vi "Any to LabVIEW data.vi"(8 "error in":errorcluster, 10 "Data Order":T2(array[cluster]), 11 "Buffer":u8[](array[numeric])) -> (0 "error out":errorcluster, 2 "Output Data":T2(array[cluster]))   [LabVIEW 2020, in "Measurement Client Wrapper.lvclass"]
uses:
  Measurement Client Wrapper.lvclass
  <vilib>/TAF/LabVIEW Measurement Client/RPC Messages/ni_measurements_v1_Type.ctl
  <vilib>/gRPC/LabVIEW gRPC Library/Server API/typeDefs/Message Element Type.ctl
  ad0f9f6a-a690-4257-9139-53c7472e02e4.vi
  5e3468d2-7d53-449c-b4e1-cc5e8415f542.vi
  a6d26e38-1f9c-4531-8e6d-7eca794b9268.vi
  6111f2b2-3cd3-499d-ba70-c96985ac6ea8.vi
  21c55018-6bd1-46ad-94e2-895e688ed211.vi
  32480346-ebdd-43b9-a875-b6da9cef7217.vi
  4be456c1-ed59-4877-98ac-649a9044a973.vi
  e11fe247-09ff-4f5c-b897-2bd6ac17fb2f.vi
  e4b28d65-13ba-4e1e-8e9f-cbb4a39d886c.vi
  6b74e1a6-e30e-492b-a672-8f47ae6b4846.vi
  c7e14ed0-4c40-453e-98d2-21eea3b9c679.vi
  6e10cc60-964f-4e3c-a26b-7e2c601abf3f.vi
  4b20a9c0-4656-4d25-ac59-f75dc05d9fa7.vi
  999d58cf-c7d1-4a48-9a2f-662ae33a0057.vi
  b2ef58c8-55fb-46b3-8ffc-837df10363ae.vi
  811a2afd-07f9-4200-a7ec-155e2e775304.vi
  83b3a3de-e939-47b1-b683-bf64c49ab1e3.vi
  2e5f1bf6-8538-4323-9d72-f5ea1c9cc5e7.vi
  afd62ca2-246d-4ad4-bf5c-cd30e0a38d2e.vi
  b36e44fd-35bf-4184-b4fe-1327aa710fa9.vi
  613c056b-bfa0-4713-9fab-606e06d1fb15.vi
  d8424940-31d6-4816-8eab-b70d00974e91.vi
  0a60d30e-f22a-4deb-b9a9-4eb16321122e.vi
  430fb88b-afb0-4053-b427-f6628c3fec79.vi
  7ca7eab8-344c-48df-b026-809a17bb004d.vi
  89faac69-16e0-4e7e-99b5-b284c15014e6.vi
  e0a13140-8de5-47f3-97ec-5164ad61690d.vi
  32ddbda6-5255-4a5b-8b1b-da880a53ef98.vi
  20ed89fe-5e49-4e0f-9c89-ad84795baeb7.vi
  a81d3560-aafc-4ad9-a891-7c5845250d01.vi
  9ad9bf5a-c2fa-470e-917f-71ccee8fcf23.vi
  b78f8f4b-0643-45f3-92be-5419717043af.vi
  e0daed00-c2e0-4d52-9c25-0b8676dbe675.vi
  <vilib>/gRPC/LabVIEW gRPC Library/Server API/Server/Get Server DLL Path.vi
  <vilib>/gRPC/LabVIEW gRPC Library/gprc-lvsupport-release.lvlib
  <vilib>/TAF/LabVIEW Measurement Client/Measurement_client-release.lvlib
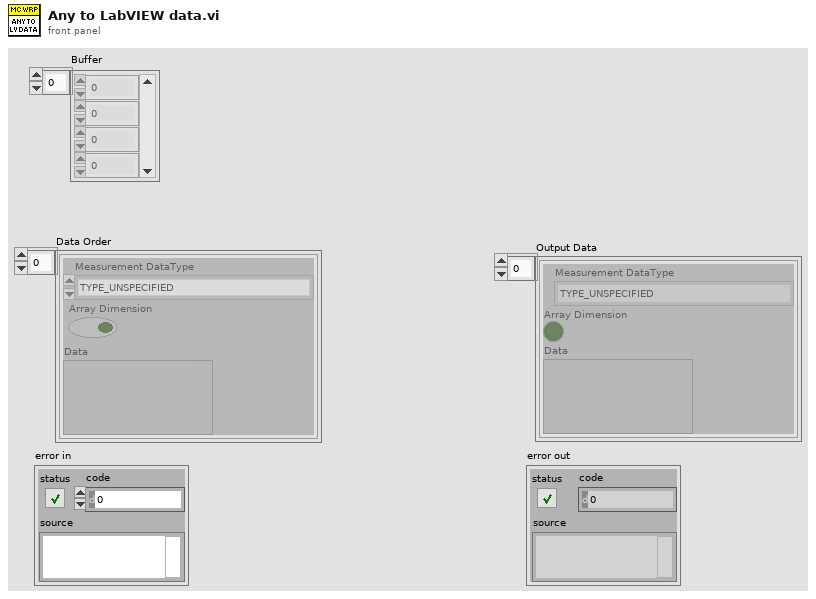
[diagram p1: front panel]
types:
  T1 = typedef "Measurement_client-release.lvlib/ni_measurements_v1_Type.ctl" = enum32{"TYPE_UNSPECIFIED", "TYPE_DOUBLE", "TYPE_FLOAT", "TYPE_INT64", "TYPE_UINT64", "TYPE_INT32", "TYPE_FIXED64", "TYPE_FIXED32", "TYPE_BOOL", "TYPE_STRING", "TYPE_GROUP", "TYPE_MESSAGE", "TYPE_BYTES", "TYPE_UINT32", "TYPE_ENUM", "TYPE_SFIXED32", "TYPE_SFIXED64", "TYPE_SINT32", "TYPE_SINT64"}
  T2 = cluster{"Measurement DataType":T1, "Array Dimension":bool, "Data":variant}[]
  T3 = typedef "gprc-lvsupport-release.lvlib/grpcId.ctl" = u64
  T4 = typedef "gprc-lvsupport-release.lvlib/Message Element Type.ctl" = enum32{"Int32Value", "FloatValue", "DoubleValue", "BoolValue", "StringValue", "MessageValue", "Int64Value", "UInt32Value", "UInt64Value", "EnumValue", "Bytes", "Fixed64", "Fixed32", "SFixed64", "SFixed32", "SInt64", "SInt32"}
  T5 = cluster{"Measurement DataType":T1, "Array Dimension":bool, "Data":variant}
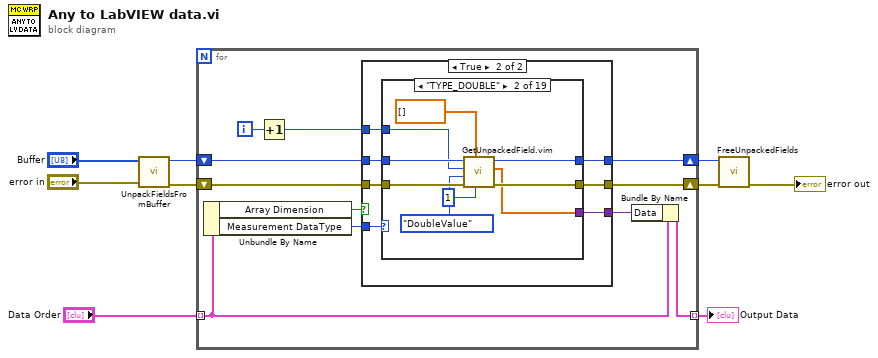
[diagram p0: block diagram]
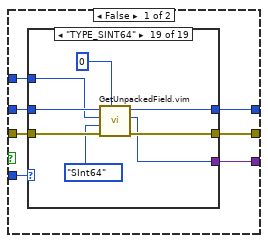
[diagram p2: hidden frame]
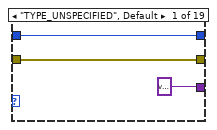
[diagram p3: hidden frame]
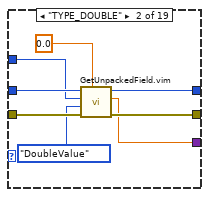
[diagram p4: hidden frame]
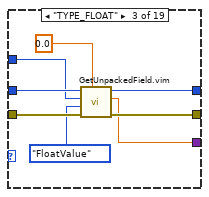
[diagram p5: hidden frame]
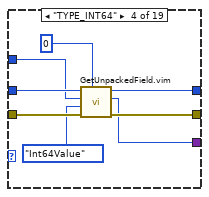
[diagram p6: hidden frame]
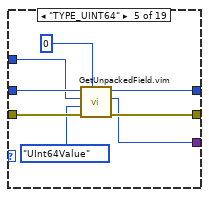
[diagram p7: hidden frame]
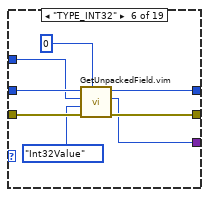
[diagram p8: hidden frame]
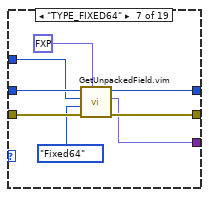
[diagram p9: hidden frame]
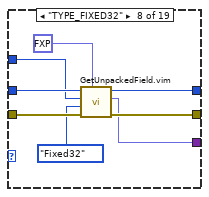
[diagram p10: hidden frame]
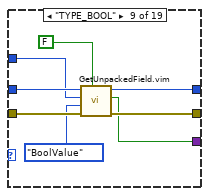
[diagram p11: hidden frame]
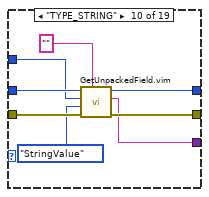
[diagram p12: hidden frame]
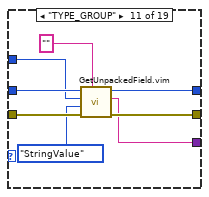
[diagram p13: hidden frame]
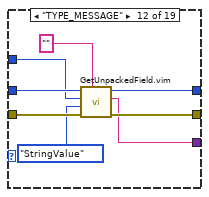
[diagram p14: hidden frame]
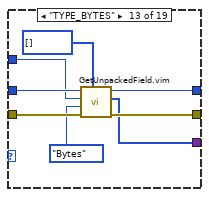
[diagram p15: hidden frame]
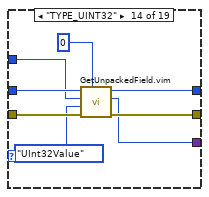
[diagram p16: hidden frame]
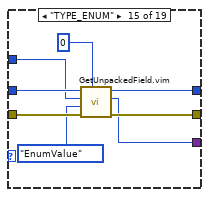
[diagram p17: hidden frame]
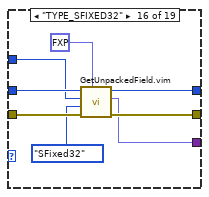
[diagram p18: hidden frame]
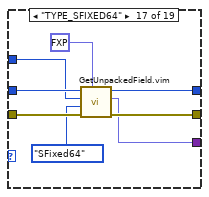
[diagram p19: hidden frame]
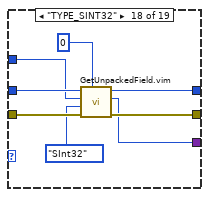
[diagram p20: hidden frame]
diagram:
  n1 = call <vilib>:"UnpackFieldsFromBuffer.vi"("error in (no error)"="error in", "Buffer"="Buffer") -> ("error out"=w8:errorcluster, "Fields Ref Out"=w9:T3)  [unwired: 8 in]
  n2 = for {
    tunnel: "Data Order" -> [w13] mode=indexing
    shift-right: [w18] -> w7
    shift-left: w9 -> [w19]
    shift-right: [w16] -> w6
    shift-left: w8 -> [w17]
    tunnel: [w11] -> w1 mode=indexing
    i -> [w15]
    n3 = Unbundle By Name(w13) -> ("Array Dimension"=w10:bool, "Measurement DataType"=w20:T1)
    n4 = Increment(x=w15) -> (x+1=w14:i32)
    n5 = case shown="True" w10 {
      tunnel: w20 -> [w27 w181]
      tunnel: w19 -> [w26 w180]
      tunnel: [w25 w179] -> w18
      tunnel: w17 -> [w24 w178]
      tunnel: [w23 w177] -> w16
      tunnel: w14 -> [w22 w176]
      tunnel: [w21 w175] -> w12
      frame False {
        n6 = case shown="\"TYPE_SINT64\"" w27 {
          tunnel: w26 -> [w30 w38 w46 w54 w62 w70 w78 w86 w94 w102 w110 w118 w126 w134 w142 w150 w158 w166 w174]
          tunnel: [w30 w36 w44 w52 w60 w68 w76 w84 w92 w100 w108 w116 w124 w132 w140 w148 w156 w164 w172] -> w25
          tunnel: w24 -> [w29 w37 w45 w53 w61 w69 w77 w85 w93 w101 w109 w117 w125 w133 w141 w149 w157 w165 w173]
          tunnel: [w29 w35 w43 w51 w59 w67 w75 w83 w91 w99 w107 w115 w123 w131 w139 w147 w155 w163 w171] -> w23
          tunnel: w22 -> [_ w33 w41 w49 w57 w65 w73 w81 w89 w97 w105 w113 w122 w130 w138 w146 w154 w162 w170]
          tunnel: [variant w31 w39 w47 w55 w63 w71 w79 w87 w95 w103 w111 w120 w128 w136 w144 w152 w160 w168] -> w21
          frame "TYPE_UNSPECIFIED", Default {
          }
          frame "TYPE_DOUBLE" {
            n7 = call "GetUnpackedField.vim"("Value"=0.0, "error in (no error)"=w37, "MessageElementType"=Message_Element_Type."DoubleValue", "protobufId"=w33, "gRPCid in"=w38) -> ("error out"=w35:errorcluster, "value"=w31:dbl, "gRPCid"=w36:u64)  [unwired: 4 in]
          }
          frame "TYPE_FLOAT" {
            n8 = call "GetUnpackedField.vim"("Value"=sgl 0.0, "error in (no error)"=w45, "MessageElementType"=Message_Element_Type."FloatValue", "protobufId"=w41, "gRPCid in"=w46) -> ("error out"=w43:errorcluster, "value"=w39:sgl, "gRPCid"=w44:u64)  [unwired: 4 in]
          }
          frame "TYPE_INT64" {
            n9 = call "GetUnpackedField.vim"("Value"=i64 0, "error in (no error)"=w53, "MessageElementType"=Message_Element_Type."Int64Value", "protobufId"=w49, "gRPCid in"=w54) -> ("error out"=w51:errorcluster, "value"=w47:i64, "gRPCid"=w52:u64)  [unwired: 4 in]
          }
          frame "TYPE_UINT64" {
            n10 = call "GetUnpackedField.vim"("Value"=u64 0, "error in (no error)"=w61, "MessageElementType"=Message_Element_Type."UInt64Value", "protobufId"=w57, "gRPCid in"=w62) -> ("error out"=w59:errorcluster, "value"=w55:u64, "gRPCid"=w60:u64)  [unwired: 4 in]
          }
          frame "TYPE_INT32" {
            n11 = call "GetUnpackedField.vim"("Value"=0, "error in (no error)"=w69, "MessageElementType"=Message_Element_Type."Int32Value", "protobufId"=w65, "gRPCid in"=w70) -> ("error out"=w67:errorcluster, "value"=w63:i32, "gRPCid"=w68:u64)  [unwired: 4 in]
          }
          frame "TYPE_FIXED64" {
            n12 = call "GetUnpackedField.vim"("Value"=fxp<+,1,1> 0.0, "error in (no error)"=w77, "MessageElementType"=Message_Element_Type."Fixed64", "protobufId"=w73, "gRPCid in"=w78) -> ("error out"=w75:errorcluster, "value"=w71:fxp<+,1,1>, "gRPCid"=w76:u64)  [unwired: 4 in]
          }
          frame "TYPE_FIXED32" {
            n13 = call "GetUnpackedField.vim"("Value"=fxp<+,1,1> 0.0, "error in (no error)"=w85, "MessageElementType"=Message_Element_Type."Fixed32", "protobufId"=w81, "gRPCid in"=w86) -> ("error out"=w83:errorcluster, "value"=w79:fxp<+,1,1>, "gRPCid"=w84:u64)  [unwired: 4 in]
          }
          frame "TYPE_BOOL" {
            n14 = call "GetUnpackedField.vim"("Value"=FALSE, "error in (no error)"=w93, "MessageElementType"=Message_Element_Type."BoolValue", "protobufId"=w89, "gRPCid in"=w94) -> ("error out"=w91:errorcluster, "value"=w87:bool, "gRPCid"=w92:u64)  [unwired: 4 in]
          }
          frame "TYPE_STRING" {
            n15 = call "GetUnpackedField.vim"("Value"="", "error in (no error)"=w101, "MessageElementType"=Message_Element_Type."StringValue", "protobufId"=w97, "gRPCid in"=w102) -> ("error out"=w99:errorcluster, "value"=w95:string, "gRPCid"=w100:u64)  [unwired: 4 in]
          }
          frame "TYPE_GROUP" {
            n16 = call "GetUnpackedField.vim"("Value"="", "error in (no error)"=w109, "MessageElementType"=Message_Element_Type."StringValue", "protobufId"=w105, "gRPCid in"=w110) -> ("error out"=w107:errorcluster, "value"=w103:string, "gRPCid"=w108:u64)  [unwired: 4 in]
          }
          frame "TYPE_MESSAGE" {
            n17 = call "GetUnpackedField.vim"("Value"="", "error in (no error)"=w117, "MessageElementType"=Message_Element_Type."StringValue", "protobufId"=w113, "gRPCid in"=w118) -> ("error out"=w115:errorcluster, "value"=w111:string, "gRPCid"=w116:u64)  [unwired: 4 in]
          }
          frame "TYPE_BYTES" {
            n18 = call "GetUnpackedField.vim"("Value"=u8[] [], "error in (no error)"=w125, "MessageElementType"=Message_Element_Type."Bytes", "protobufId"=w122, "gRPCid in"=w126) -> ("error out"=w123:errorcluster, "value"=w120:u8[], "gRPCid"=w124:u64)  [unwired: 4 in]
          }
          frame "TYPE_UINT32" {
            n19 = call "GetUnpackedField.vim"("Value"=u32 0, "error in (no error)"=w133, "MessageElementType"=Message_Element_Type."UInt32Value", "protobufId"=w130, "gRPCid in"=w134) -> ("error out"=w131:errorcluster, "value"=w128:u32, "gRPCid"=w132:u64)  [unwired: 4 in]
          }
          frame "TYPE_ENUM" {
            n20 = call "GetUnpackedField.vim"("Value"=0, "error in (no error)"=w141, "MessageElementType"=Message_Element_Type."EnumValue", "protobufId"=w138, "gRPCid in"=w142) -> ("error out"=w139:errorcluster, "value"=w136:i32, "gRPCid"=w140:u64)  [unwired: 4 in]
          }
          frame "TYPE_SFIXED32" {
            n21 = call "GetUnpackedField.vim"("Value"=fxp<+,1,1> 0.0, "error in (no error)"=w149, "MessageElementType"=Message_Element_Type."SFixed32", "protobufId"=w146, "gRPCid in"=w150) -> ("error out"=w147:errorcluster, "value"=w144:fxp<+,1,1>, "gRPCid"=w148:u64)  [unwired: 4 in]
          }
          frame "TYPE_SFIXED64" {
            n22 = call "GetUnpackedField.vim"("Value"=fxp<+,1,1> 0.0, "error in (no error)"=w157, "MessageElementType"=Message_Element_Type."SFixed64", "protobufId"=w154, "gRPCid in"=w158) -> ("error out"=w155:errorcluster, "value"=w152:fxp<+,1,1>, "gRPCid"=w156:u64)  [unwired: 4 in]
          }
          frame "TYPE_SINT32" {
            n23 = call "GetUnpackedField.vim"("Value"=0, "error in (no error)"=w165, "MessageElementType"=Message_Element_Type."SInt32", "protobufId"=w162, "gRPCid in"=w166) -> ("error out"=w163:errorcluster, "value"=w160:i32, "gRPCid"=w164:u64)  [unwired: 4 in]
          }
          frame "TYPE_SINT64" {
            n24 = call "GetUnpackedField.vim"("Value"=i64 0, "error in (no error)"=w173, "MessageElementType"=Message_Element_Type."SInt64", "protobufId"=w170, "gRPCid in"=w174) -> ("error out"=w171:errorcluster, "value"=w168:i64, "gRPCid"=w172:u64)  [unwired: 4 in]
          }
        }
      }
      frame True {
        n25 = case shown="\"TYPE_DOUBLE\"" w181 {
          tunnel: w180 -> [w184 w193 w202 w211 w220 w229 w238 w247 w256 w265 w268 w271 w274 w283 w292 w301 w310 w319 w328]
          tunnel: [w184 w191 w200 w209 w218 w227 w236 w245 w254 w263 w268 w271 w274 w281 w290 w299 w308 w317 w326] -> w179
          tunnel: w178 -> [w183 w192 w201 w210 w219 w228 w237 w246 w255 w264 w267 w270 w273 w282 w291 w300 w309 w318 w327]
          tunnel: [w183 w190 w199 w208 w217 w226 w235 w244 w253 w262 w267 w270 w273 w280 w289 w298 w307 w316 w325] -> w177
          tunnel: w176 -> [_ w189 w198 w207 w216 w225 w234 w243 w252 w261 _ _ _ w279 w288 w297 w306 w315 w324]
          tunnel: [variant w187 w196 w205 w214 w223 w232 w241 w250 w259 variant ("value") variant ("value") variant ("value") w277 w286 w295 w304 w313 w322] -> w175
          frame "TYPE_UNSPECIFIED", Default {
          }
          frame "TYPE_DOUBLE" {
            n26 = call "GetUnpackedField.vim"("isRepeated"=1, "Value"=dbl[] [], "error in (no error)"=w192, "MessageElementType"=Message_Element_Type."DoubleValue", "protobufId"=w189, "gRPCid in"=w193) -> ("error out"=w190:errorcluster, "value"=w187:dbl[], "gRPCid"=w191:u64)  [unwired: 3 in]
          }
          frame "TYPE_FLOAT" {
            n27 = call "GetUnpackedField.vim"("isRepeated"=1, "Value"=sgl[] [], "error in (no error)"=w201, "MessageElementType"=Message_Element_Type."FloatValue", "protobufId"=w198, "gRPCid in"=w202) -> ("error out"=w199:errorcluster, "value"=w196:sgl[], "gRPCid"=w200:u64)  [unwired: 3 in]
          }
          frame "TYPE_INT64" {
            n28 = call "GetUnpackedField.vim"("isRepeated"=1, "Value"=i64[] [], "error in (no error)"=w210, "MessageElementType"=Message_Element_Type."Int64Value", "protobufId"=w207, "gRPCid in"=w211) -> ("error out"=w208:errorcluster, "value"=w205:i64[], "gRPCid"=w209:u64)  [unwired: 3 in]
          }
          frame "TYPE_UINT64" {
            n29 = call "GetUnpackedField.vim"("isRepeated"=1, "Value"=u64[] [], "error in (no error)"=w219, "MessageElementType"=Message_Element_Type."UInt64Value", "protobufId"=w216, "gRPCid in"=w220) -> ("error out"=w217:errorcluster, "value"=w214:u64[], "gRPCid"=w218:u64)  [unwired: 3 in]
          }
          frame "TYPE_INT32" {
            n30 = call "GetUnpackedField.vim"("isRepeated"=1, "Value"=i32[] [], "error in (no error)"=w228, "MessageElementType"=Message_Element_Type."Int32Value", "protobufId"=w225, "gRPCid in"=w229) -> ("error out"=w226:errorcluster, "value"=w223:i32[], "gRPCid"=w227:u64)  [unwired: 3 in]
          }
          frame "TYPE_FIXED64" {
            n31 = call "GetUnpackedField.vim"("isRepeated"=1, "Value"=fxp<+,1,1>[] [], "error in (no error)"=w237, "MessageElementType"=Message_Element_Type."Fixed64", "protobufId"=w234, "gRPCid in"=w238) -> ("error out"=w235:errorcluster, "value"=w232:fxp<+,1,1>[], "gRPCid"=w236:u64)  [unwired: 3 in]
          }
          frame "TYPE_FIXED32" {
            n32 = call "GetUnpackedField.vim"("isRepeated"=1, "Value"=u32[] [], "error in (no error)"=w246, "MessageElementType"=Message_Element_Type."Fixed32", "protobufId"=w243, "gRPCid in"=w247) -> ("error out"=w244:errorcluster, "value"=w241:u32[], "gRPCid"=w245:u64)  [unwired: 3 in]
          }
          frame "TYPE_BOOL" {
            n33 = call "GetUnpackedField.vim"("isRepeated"=1, "Value"=bool[] [], "error in (no error)"=w255, "MessageElementType"=Message_Element_Type."BoolValue", "protobufId"=w252, "gRPCid in"=w256) -> ("error out"=w253:errorcluster, "value"=w250:bool[], "gRPCid"=w254:u64)  [unwired: 3 in]
          }
          frame "TYPE_STRING" {
            n34 = call "GetUnpackedField.vim"("isRepeated"=1, "Value"=string[] [], "error in (no error)"=w264, "MessageElementType"=Message_Element_Type."StringValue", "protobufId"=w261, "gRPCid in"=w265) -> ("error out"=w262:errorcluster, "value"=w259:string[], "gRPCid"=w263:u64)  [unwired: 3 in]
          }
          frame "TYPE_GROUP" {
          }
          frame "TYPE_MESSAGE" {
          }
          frame "TYPE_BYTES" {
          }
          frame "TYPE_UINT32" {
            n35 = call "GetUnpackedField.vim"("isRepeated"=1, "Value"=u32[] [], "error in (no error)"=w282, "MessageElementType"=Message_Element_Type."UInt32Value", "protobufId"=w279, "gRPCid in"=w283) -> ("error out"=w280:errorcluster, "value"=w277:u32[], "gRPCid"=w281:u64)  [unwired: 3 in]
          }
          frame "TYPE_ENUM" {
            n36 = call "GetUnpackedField.vim"("isRepeated"=1, "Value"=i32[] [], "error in (no error)"=w291, "MessageElementType"=Message_Element_Type."EnumValue", "protobufId"=w288, "gRPCid in"=w292) -> ("error out"=w289:errorcluster, "value"=w286:i32[], "gRPCid"=w290:u64)  [unwired: 3 in]
          }
          frame "TYPE_SFIXED32" {
            n37 = call "GetUnpackedField.vim"("isRepeated"=1, "Value"=fxp<+,1,1>[] [], "error in (no error)"=w300, "MessageElementType"=Message_Element_Type."SFixed32", "protobufId"=w297, "gRPCid in"=w301) -> ("error out"=w298:errorcluster, "value"=w295:fxp<+,1,1>[], "gRPCid"=w299:u64)  [unwired: 3 in]
          }
          frame "TYPE_SFIXED64" {
            n38 = call "GetUnpackedField.vim"("isRepeated"=1, "Value"=fxp<+,1,1>[] [], "error in (no error)"=w309, "MessageElementType"=Message_Element_Type."SFixed64", "protobufId"=w306, "gRPCid in"=w310) -> ("error out"=w307:errorcluster, "value"=w304:fxp<+,1,1>[], "gRPCid"=w308:u64)  [unwired: 3 in]
          }
          frame "TYPE_SINT32" {
            n39 = call "GetUnpackedField.vim"("isRepeated"=1, "Value"=i32[] [], "error in (no error)"=w318, "MessageElementType"=Message_Element_Type."SInt32", "protobufId"=w315, "gRPCid in"=w319) -> ("error out"=w316:errorcluster, "value"=w313:i32[], "gRPCid"=w317:u64)  [unwired: 3 in]
          }
          frame "TYPE_SINT64" {
            n40 = call "GetUnpackedField.vim"("isRepeated"=1, "Value"=i64[] [], "error in (no error)"=w327, "MessageElementType"=Message_Element_Type."SInt64", "protobufId"=w324, "gRPCid in"=w328) -> ("error out"=w325:errorcluster, "value"=w322:i64[], "gRPCid"=w326:u64)  [unwired: 3 in]
          }
        }
      }
    }
    n41 = Bundle By Name(cluster=w13, "Data"=w12) -> (w11:T5)
  }
  "Output Data" <- w1
  n42 = call <vilib>:"FreeUnpackedFields.vi"("error in (no error)"=w6, "Unpacked Fields ID"=w7) -> ("error out"=→"error out":errorcluster)  [unwired: 9 in]
